vi "PKYK_State_Queue_read.vi"(6 "Img. In":picture[](array[picture]), 7 "PKYK In":T4[](array[typedef]), 8 "error in (no error)":errorcluster, 9 "Ref in":T1={"MS SQL Connection"=refnum, "UDL File"=path "", "Time"="", "DCODE"="", "WIP+1"=0, "MC No?"=0, "POKAYOKE?"=FALSE, "Expected Result"="", "Result [Status]"="", "Clock"=0.0, "RFID"="", "WIP Queue"=refnum, "TS Parameter"={"ProfitCenterCode"="", "LineCode"="", "WorkOrderNumber"="", "Model"="", "Model_with_Prefix"="", "VendorCode"="", "SetParameterDateCode"="", "PokaYoke"=0, "Target"=1, "Live_DateCode"="", "CustomerPartNumber"="", "Hand"="", "sBarcode"=FALSE, "FCA"=0, "Ent_Stamp"=timestamp(0 s since 1904-01-01), "STS_CD"=0.0}, "Data_Queue"=[], "RFID Serial No."=""} {"TS Parameter"."FCA" format="%01d"; "TS Parameter"."Target" min=1 max=100000; "TS Parameter"."PokaYoke" min=0 max=1}, 10 "State In":T8, 11 "Queue In":refnum<queue>) -> (0 "error out":errorcluster, 1 "PKYK_Data Out":T4, 2 "PKYK_Data":cluster{"PKYK 1":picture, "PKYK 1":picture}, 3 "Queue out":refnum<queue>, 4 "Img. Out":picture[](array[picture]), 5 "PKYK Out":T4[](array[typedef]))   [LabVIEW 2020]
uses:
  Controls/PKYK_qData.ctl
  Controls/Poka_Status.ctl
  Controls/PKYK_Barcode_Status.ctl
  Controls/PKYK_Status.ctl
  Controls/WIP_State.ctl
  Controls/TD SQL.ctl
  <vilib>/addons/database/Connection.llb/Conn ObjectReference.ctl
  Controls/TS_Parameter.ctl
  MS SQL/MS_Global.vi
  <vilib>/addons/database/NI_Database_API.lvlib
panel:
  in  "value":bool
  out "PKYK_Data 2":picture
  out "PKYK_Data 1":picture
  in  "PKYK_Data In":T4
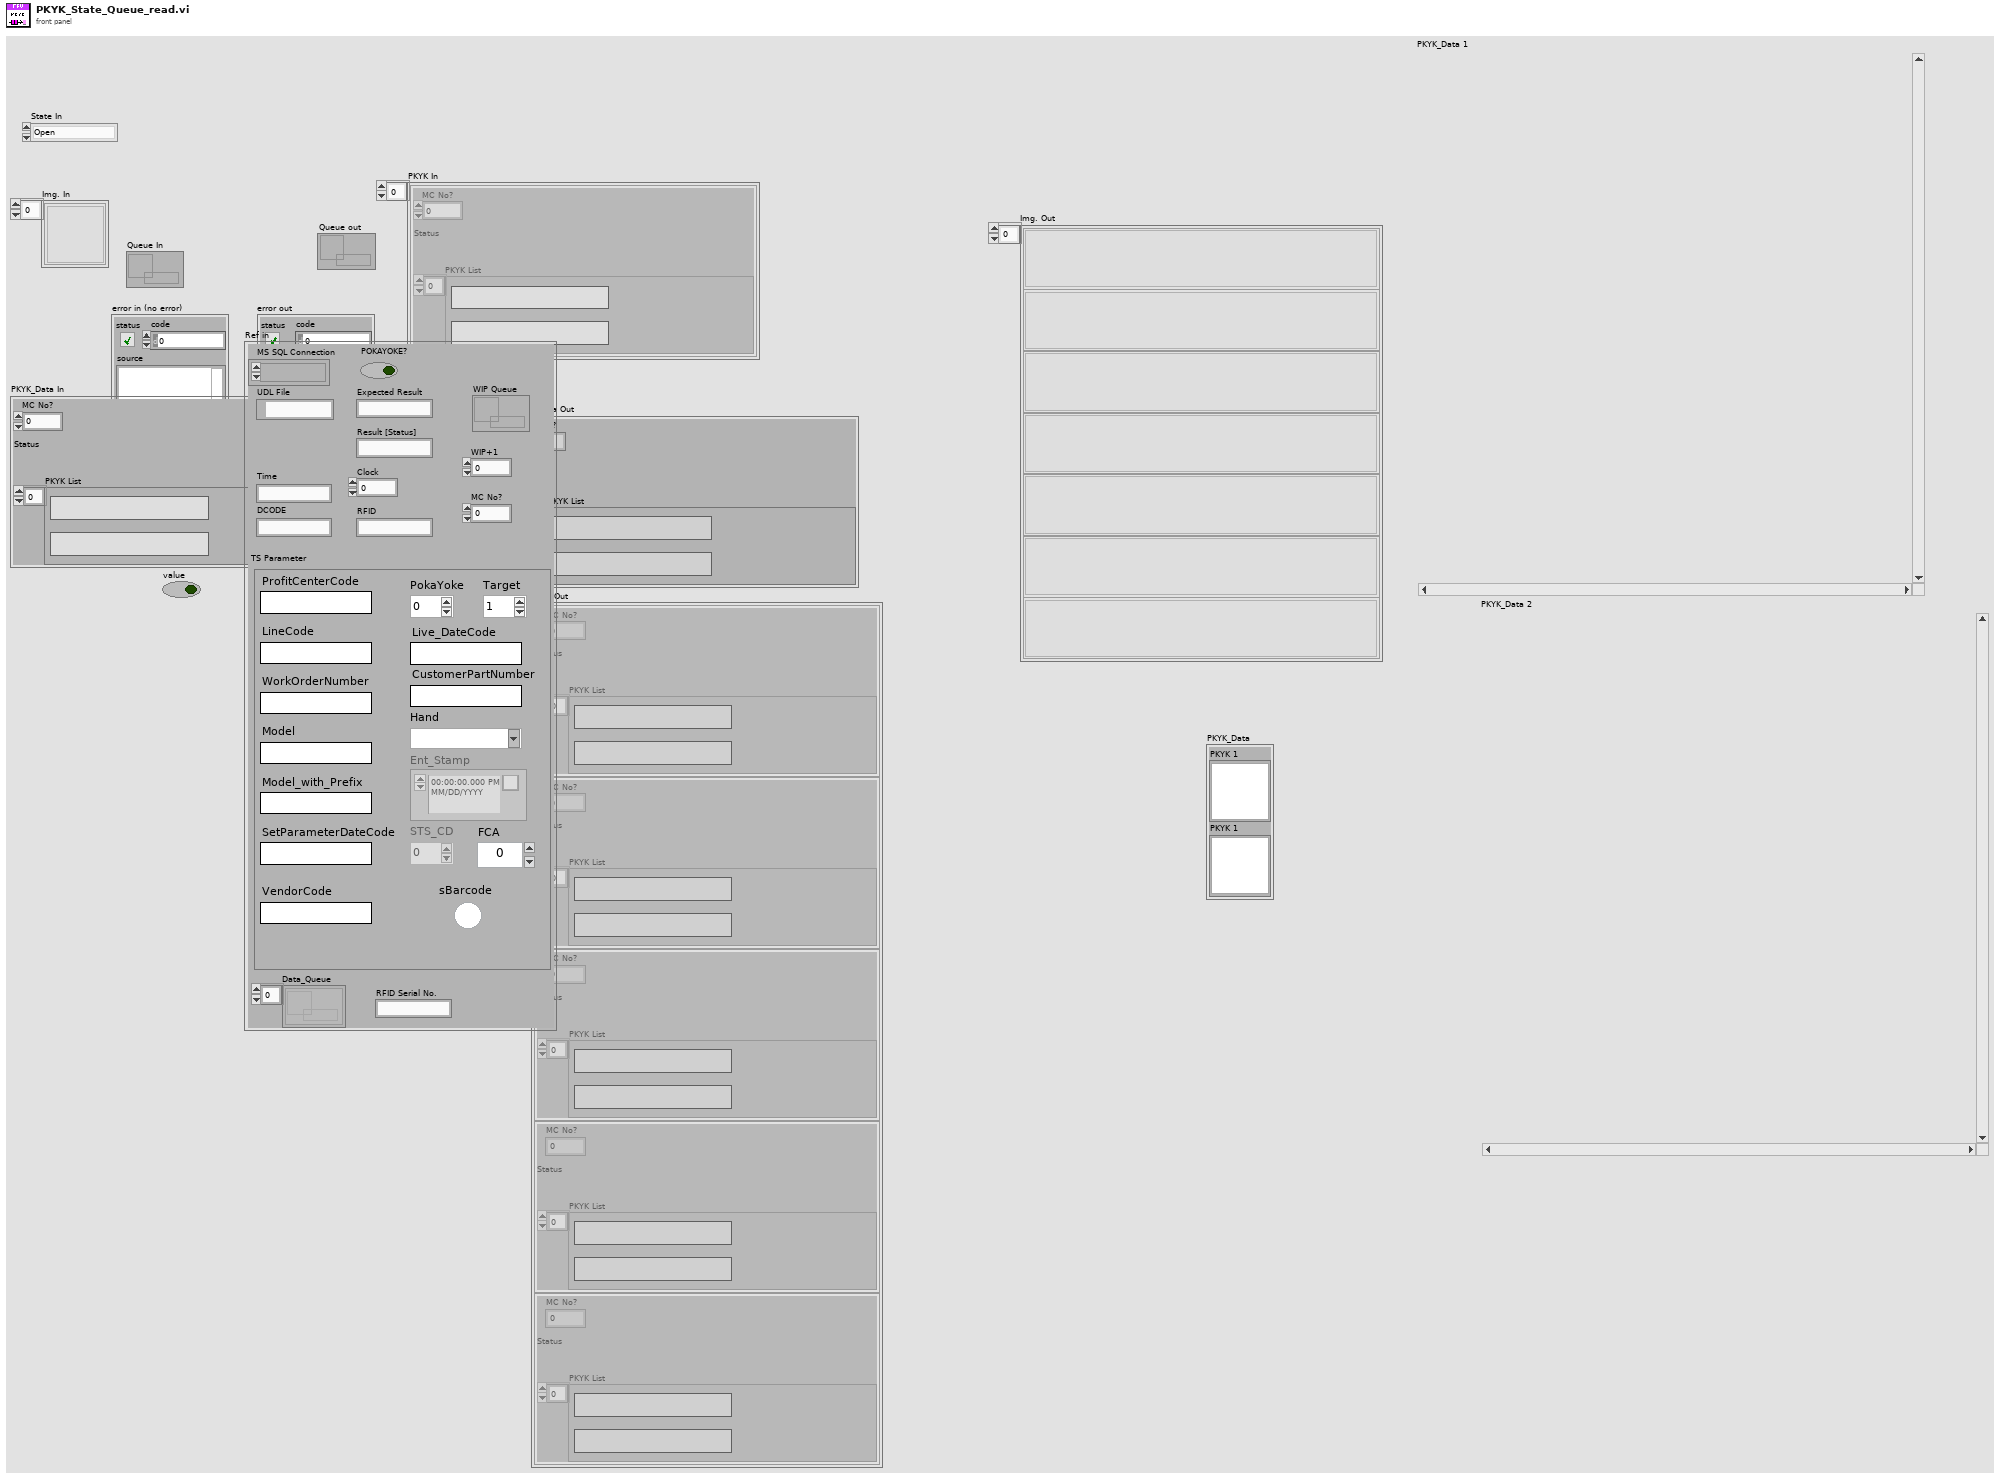
[diagram p1: front panel]
types:
  T1 = typedef "TD SQL.ctl" = cluster{"MS SQL Connection":T2, "UDL File":path, "Time":string, "DCODE":string, "WIP+1":i64, "MC No?":i32, "POKAYOKE?":bool, "Expected Result":string, "Result [Status]":string, "Clock":dbl, "RFID":string, "WIP Queue":refnum<queue>, "TS Parameter":T3, "Data_Queue":refnum<queue>[], "RFID Serial No.":string}
  T2 = typedef "NI_Database_API.lvlib/Conn ObjectReference.ctl" = refnum<k1>
  T3 = typedef "TS_Parameter.ctl" = cluster{"ProfitCenterCode":string, "LineCode":string, "WorkOrderNumber":string, "Model":string, "Model_with_Prefix":string, "VendorCode":string, "SetParameterDateCode":string, "PokaYoke":i32, "Target":i32, "Live_DateCode":string, "CustomerPartNumber":string, "Hand":string, "sBarcode":bool, "FCA":i32, "Ent_Stamp":timestamp, "STS_CD":dbl}
  T4 = typedef "PKYK_qData.ctl" = cluster{"MC No?":i32, "Status":T5, "PKYK List":T6[]}
  T5 = typedef "Poka_Status.ctl" = u16
  T6 = typedef "PKYK_Barcode_Status.ctl" = cluster{"RFID Written Last":string, "Result":T7, "Exp. Result":T7}
  T7 = typedef "PKYK_Status.ctl" = u16
  T8 = typedef "WIP_State.ctl" = enum16{"Open", "Read", "Write", "Read WIP", "Flush", "Close"}
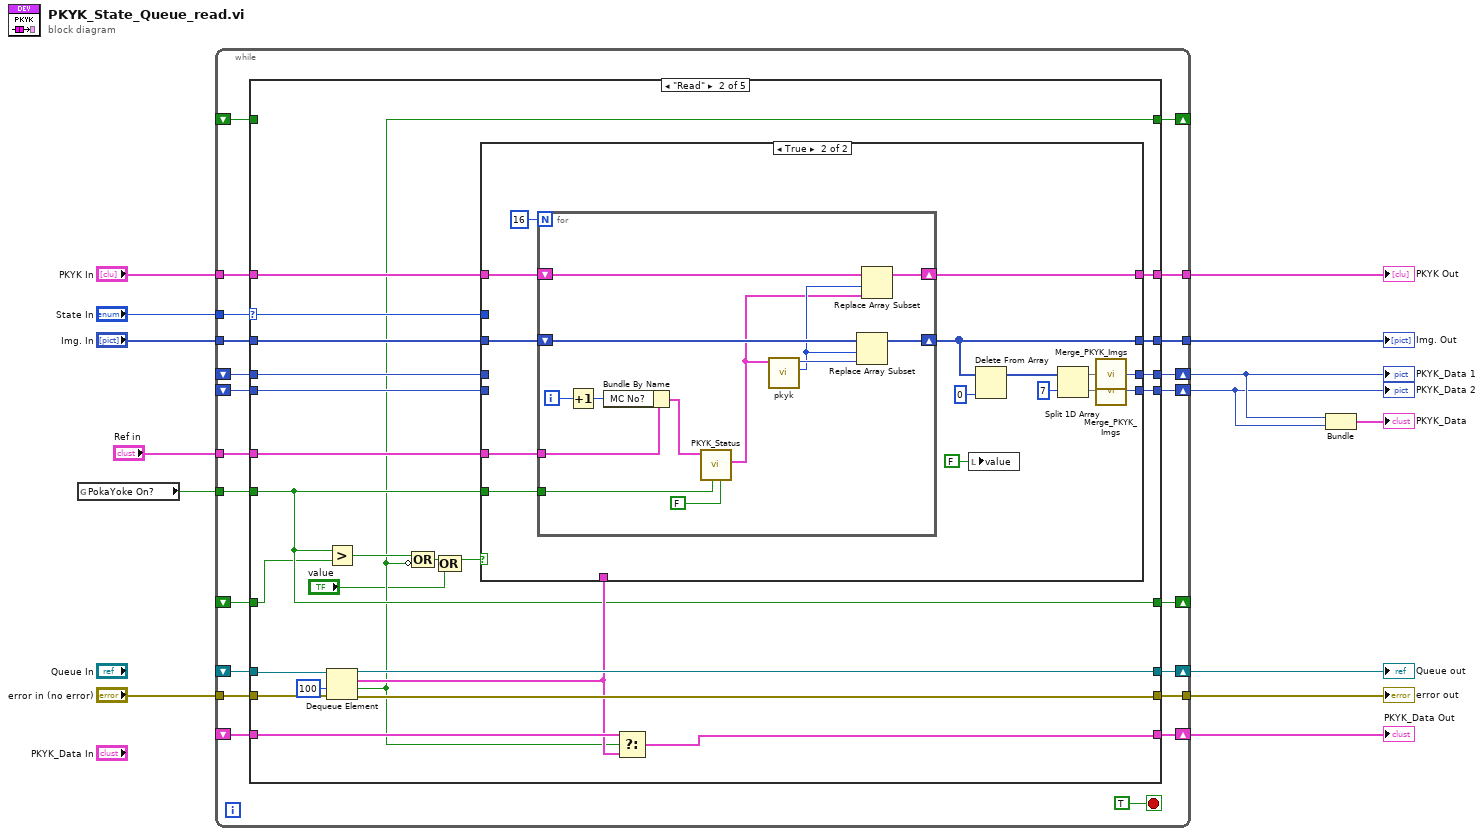
[diagram p0: block diagram]
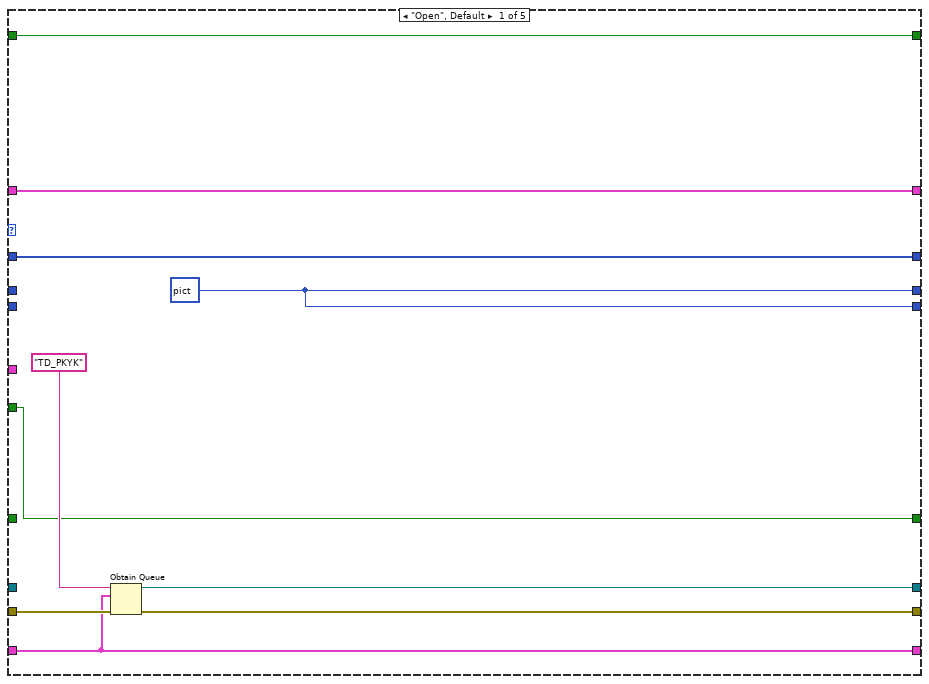
[diagram p2: hidden frame]
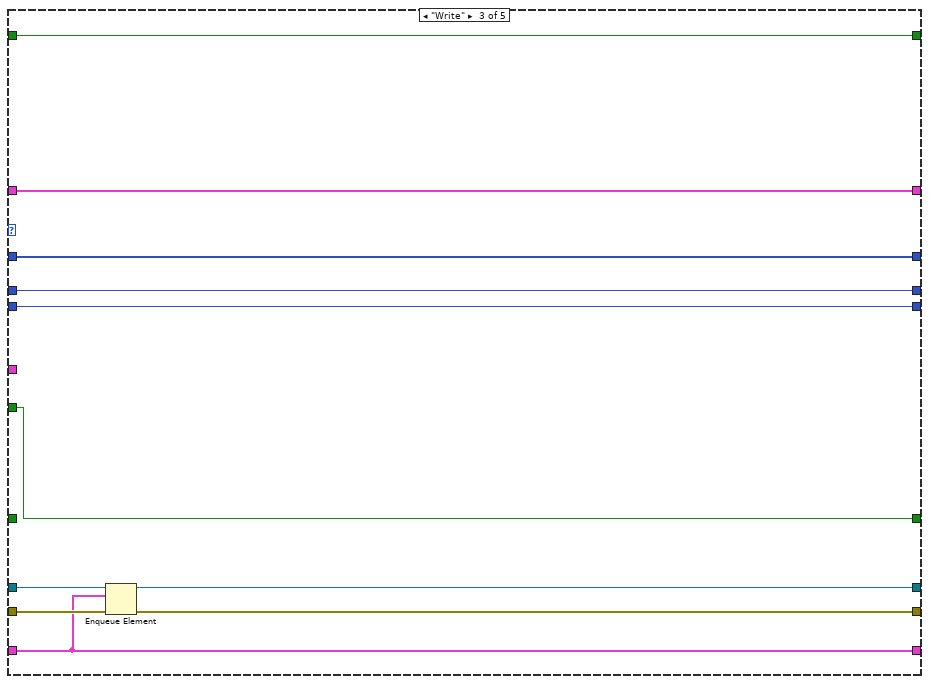
[diagram p4: hidden frame]
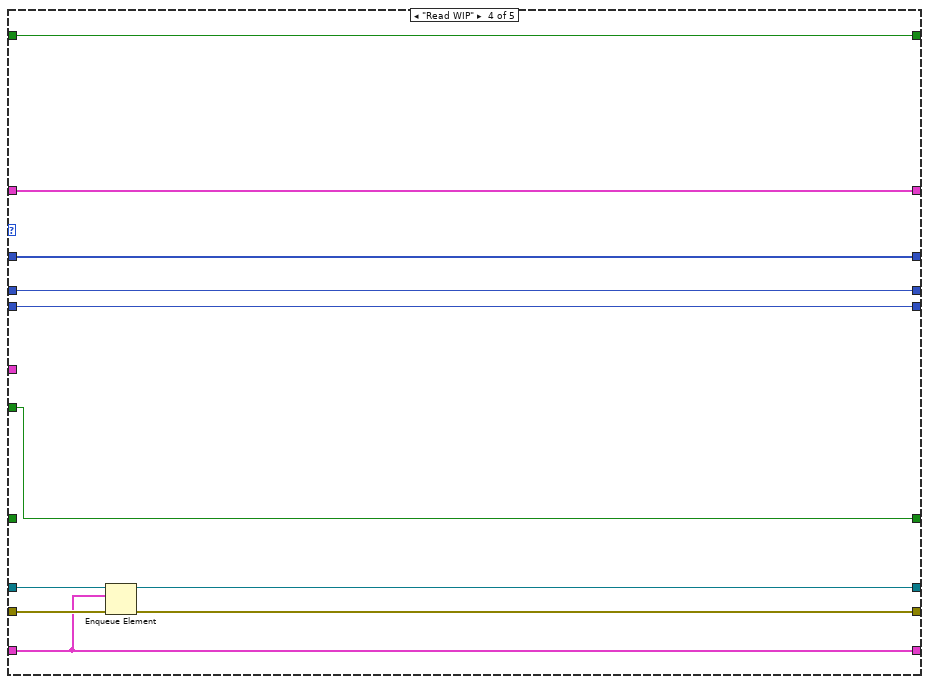
[diagram p5: hidden frame]
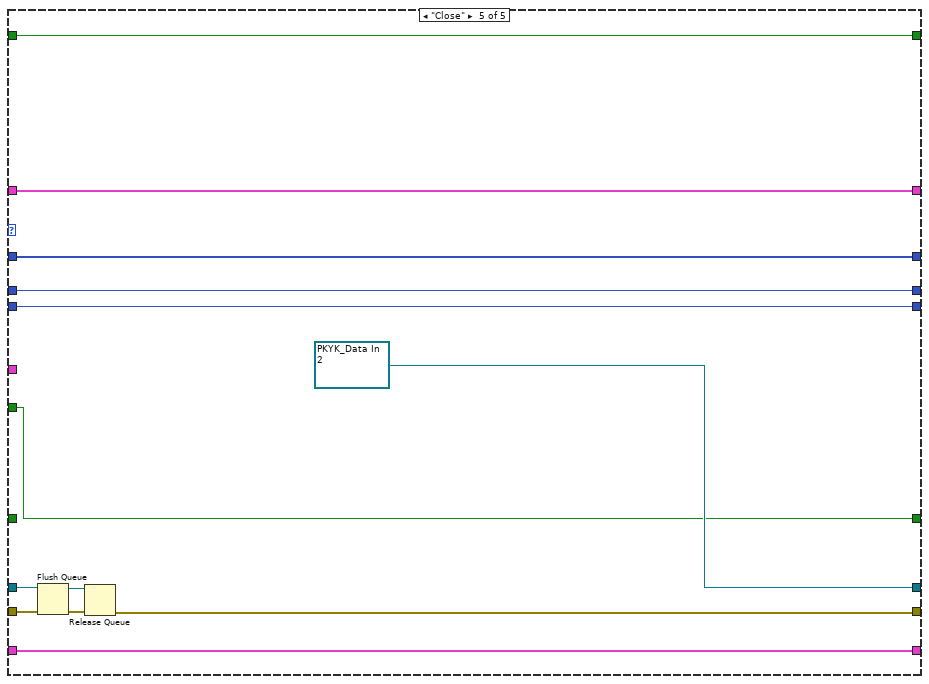
[diagram p6: hidden frame]
diagram:
  n1 = global read "MS_Global.vi" "PokaYoke On?"() -> (w1:bool)
  n2 = while {
    tunnel: "State In" -> [w32]
    shift-right: [w35] -> w13
    shift-left: _ -> [w31]
    tunnel: "error in (no error)" -> [w34]
    tunnel: [w36] -> w14
    shift-right: [w29] -> w10
    shift-left: _ -> [w30]
    tunnel: "PKYK In" -> [w28]
    tunnel: [w27] -> w8
    shift-right: [w26] -> _
    shift-left: _ -> [w25]
    tunnel: "Img. In" -> [w24]
    tunnel: [w23] -> w6
    shift-right: [w22] -> w5
    shift-left: _ -> [w21]
    shift-right: [w19] -> w4
    shift-left: _ -> [w20]
    tunnel: "Ref in" -> [w18]
    shift-right: [w17] -> _
    shift-left: _ -> [w16]
    tunnel: w1 -> [w15]
    stop <- TRUE stop-if-true
    n3 = case shown="\"Read\"" w32 {
      selector: w32 -> [_ w62 _ _ _]
      tunnel: [w46 w69 w111 w122 w134] -> w36
      tunnel: [w45 w68 w112 w123 refnum<queue> refnum ("Queue In")] -> w35
      tunnel: w34 -> [w43 w71 w113 w124 w138]
      tunnel: w31 -> [_ w70 w114 w125 w137]
      tunnel: [w42 w67 w110 w121 w132] -> w29
      tunnel: w30 -> [w42 w66 w110 w121 w132]
      tunnel: w28 -> [w41 w65 w109 w120 w131]
      tunnel: [w41 w63 w109 w120 w131] -> w27
      tunnel: [w40 w49 w108 w119 w130] -> w26
      tunnel: w25 -> [w40 _ w108 w119 w130]
      tunnel: w24 -> [w39 w61 w107 w118 w129]
      tunnel: [w39 w60 w107 w118 w129] -> w23
      tunnel: [w38 w59 w106 w117 w128] -> w22
      tunnel: w21 -> [_ w58 w106 w117 w128]
      tunnel: w20 -> [_ w56 w105 w116 w127]
      tunnel: [w38 w57 w105 w116 w127] -> w19
      tunnel: w18 -> [_ w55 _ _ _]
      tunnel: [w37 w54 w104 w115 w126] -> w17
      tunnel: w16 -> [_ w53 _ _ _]
      tunnel: w15 -> [w37 w54 w104 w115 w126]
      frame "Open", Default {
        w38 = picture data[5B] ("PKYK")
        n4 = Obtain Queue(name (unnamed)="TD_PKYK", element data type=w42, error in (no error)=w43) -> (queue out=w45:refnum<queue>, error out=w46:errorcluster)  [unwired: 2 in, 1 out]
      }
      frame "Read" {
        n5 = Greater?(x=w54, y=w53) -> (0:w52:bool)
        n6 = Dequeue Element(queue=w70, timeout in ms (-1)=100, error in (no error)=w71) -> (queue out=w68:refnum<queue>, element=w64:T4, timed out?=w49:bool, error out=w69:errorcluster)
        n7 = Compound Arithmetic op=OR(w52, invert w49) -> (w50:bool)
        n8 = Compound Arithmetic op=OR(w50, "value") -> (w48:bool)
        n9 = case shown="True" w48 {
          tunnel: w65 -> [w75 w90]
          tunnel: w64 -> [_ _]
          tunnel: [w75 w89] -> w63
          tunnel: w62 -> [_ _]
          tunnel: w61 -> [w74 w88]
          tunnel: [w74 w82] -> w60
          tunnel: [w73 w87] -> w59
          tunnel: w58 -> [w73 _]
          tunnel: [w72 w86] -> w57
          tunnel: w56 -> [w72 _]
          tunnel: w54 -> [_ w79]
          tunnel: w55 -> [_ w78]
          frame False {
          }
          frame True {
            n10 = for {
              N: 16 -> [_]
              tunnel: w79 -> [w97]
              tunnel: w78 -> [w96]
              shift-right: [w102] -> w89
              shift-left: w90 -> [w103]
              shift-right: [w98] -> w82
              shift-left: w88 -> [w101]
              i -> [w93]
              n11 = Increment(x=w93) -> (x+1=w92:i32)
              n12 = Bundle By Name(cluster=w96, "MC No?"=w92) -> (w94:T1)
              n13 = call "PKYK_Status.vi"("QUpdate"=FALSE, "PokaYoke?"=w97, "Ref in"=w94) -> ("PKYK_Data Out"=w95:T4)  [unwired: 5 in, 3 out]
              n14 = call "pkyk.vi"("New PKYK"=w95) -> ("MC No?"=w99:i32, "PKYK"=w100:picture)  [unwired: 8 in, 1 out]
              n15 = Replace Array Subset(array=w101, new element=w100, index=w99) -> (w98:picture[])
              n16 = Replace Array Subset(array=w103, new element=w95, index=w99) -> (w102:T4[])
            }
            n17 = local write "value"(FALSE ("value")) -> ()
            n18 = Delete From Array(array=w82, index=0) -> (array with subset deleted=w81:picture[])  [unwired: 1 in, 1 out]
            n19 = Split 1D Array(array=w81, index=7) -> (first subarray=w85:picture[], second subarray=w84:picture[])
            n20 = call "Merge_PKYK_Imgs.vi"("Img. In"=w85) -> ("PKYK 1"=w87:picture)
            n21 = call "Merge_PKYK_Imgs.vi"("Img. In"=w84) -> ("PKYK 1"=w86:picture)
          }
        }
        n22 = Select(t=w66, s=w49, f=w64) -> (s? t:f=w67:T4)
      }
      frame "Write" {
        n23 = Enqueue Element(queue=w114, element=w110, error in (no error)=w113) -> (queue out=w112:refnum<queue>, error out=w111:errorcluster)  [unwired: 1 in, 1 out]
      }
      frame "Read WIP" {
        n24 = Enqueue Element(queue=w125, element=w121, error in (no error)=w124) -> (queue out=w123:refnum<queue>, error out=w122:errorcluster)  [unwired: 1 in, 1 out]
      }
      frame "Close" {
        n25 = Flush Queue(queue=w137, error in (no error)=w138) -> (queue out=w135:refnum<queue>, error out=w136:errorcluster)  [unwired: 1 out]
        n26 = Release Queue(queue=w135, error in (no error)=w136) -> (error out=w134:errorcluster)  [unwired: 1 in, 2 out]
      }
    }
  }
  "error out" <- w14
  "Queue out" <- w13
  "PKYK_Data Out" <- w10
  "PKYK Out" <- w8
  "Img. Out" <- w6
  "PKYK_Data 1" <- w5
  "PKYK_Data 2" <- w4
  n27 = Bundle("PKYK 1"=w5, "PKYK 1"=w4) -> (→"PKYK_Data":cluster{"PKYK 1":picture, "PKYK 1":picture})  [unwired: 1 in]
